vi "Sample_InputImpedance.vi"() -> ()   [LabVIEW 2013]
doc: "This samples demonstrates how to sample a finite waveform."
uses:
  <userlib>/ArtScope/Trigger/ArtScope_ConfigureTriggerSoftWare.vi
  <userlib>/ArtScope/Fetch/ArtScope_FetchBinary8.vi
  <userlib>/ArtScope/_SubVI/ArtScope_ArrayByChannel_U8.vi
panel:
  in  "bandwidth":i32(ring) items=["All"=-1, "Default"=0, "100M"=1, "20M"=2]
  in  "reference position":dbl
  in  "num samples":i32=1000
  in  "offset(mV)":i32
  in  "range(Vpp)":i32(ring) items=["20V", "10V", "2V", "40V", "16V", "8V", "4V", "1.6V", "800m", "400m", "160m", "80m", "40m"]
  in  "Stop":bool
  in  "input impendance":i32(ring) items=["1MΩ", "50Ω"]
  out "waveform":u8[][](graph)
  out "error out":errorcluster
  in  "timeout(s)":dbl=10.0
  in  "min record length":i32=1000
  in  "min sample rate":dbl=8000000.0
  in  "coupling":i32(ring) items=["DC", "AC"]
  in  "channel name":string="0"
  in  "resource name":string="Dev1"
  # "Vertical"
  # "Horizontal"
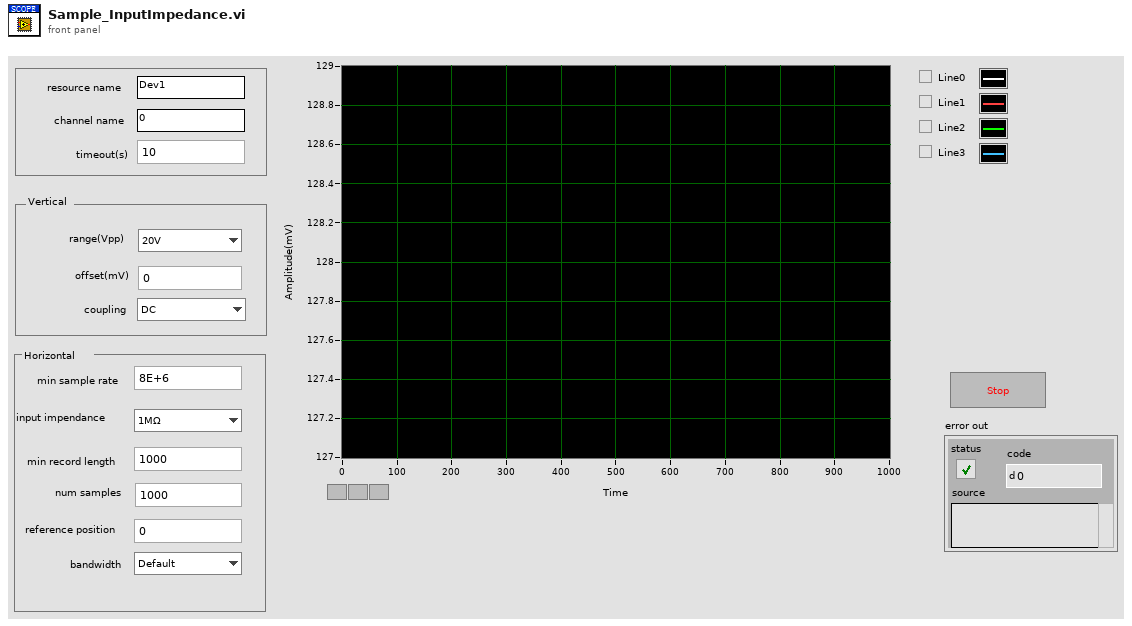
[diagram p1: front panel]
types:
  T1 = cluster{"fLSB":cluster{dbl, dbl, dbl, dbl, dbl, dbl, dbl, dbl}, "RangeValue":cluster{dbl, dbl, dbl, dbl, dbl, dbl, dbl, dbl}, "wMaxLSB":u32, "TriggerMode":i32, "sampLengthPerChan":u32, "pAvailSampsPoints":u32, "channelCount":i32}
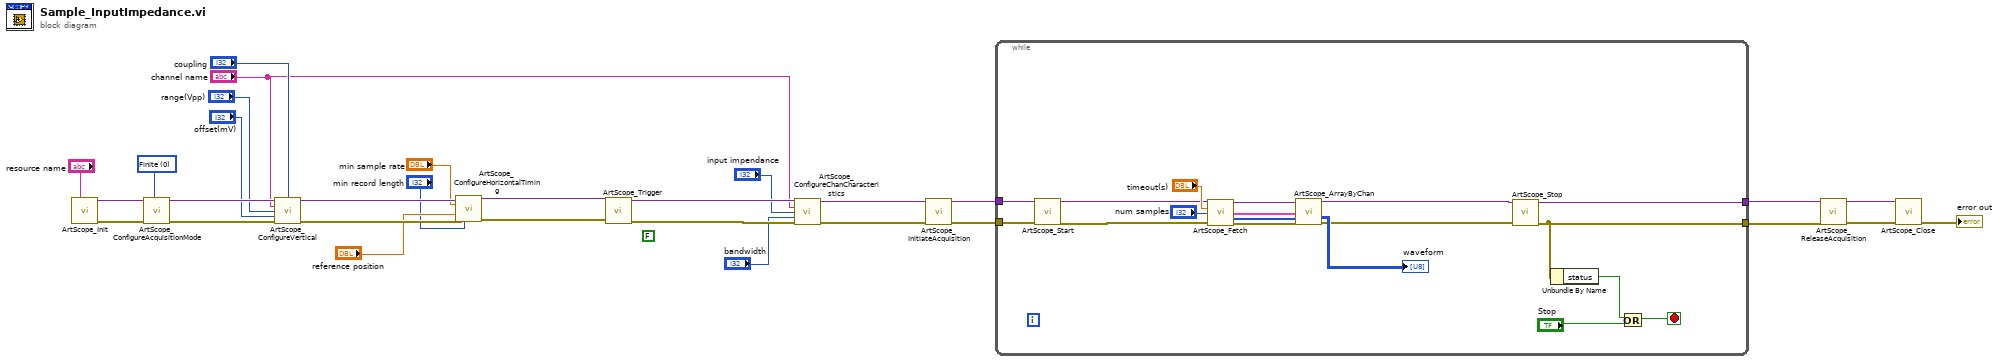
[diagram p0: block diagram]
diagram:
  (unwired) FALSE ("TrigOutEnable")
  w21 = 0 items=["Finite", "Continuous"] ("AcuqMode")
  n1 = call <userlib>:"ArtScope_Init.vi"("task name"="resource name") -> ("task handle"=w22:variant, "error out"=w23:errorcluster)  [unwired: 13 in]
  n2 = call <userlib>:"ArtScope_ConfigureAcquisitionMode.vi"("task handle"=w22, "acquisition mode"=w21, "error in (no error)"=w23) -> ("task handle"=w20:variant, "error out"=w24:errorcluster)  [unwired: 11 in]
  n3 = call <userlib>:"ArtScope_ConfigureVertical.vi"("task handle"=w20, "coupling"="coupling", "channels"="channel name", "range(Vpp)"="range(Vpp)", "offset"="offset(mV)", "error in (no error)"=w24) -> ("task handle"=w28:variant, "error out"=w27:errorcluster)  [unwired: 8 in]
  n4 = call <userlib>:"ArtScope_ConfigureHorizontalTiming.vi"("task handle"=w28, "min sample rate"="min sample rate", "reference position"="reference position", "error in (no error)"=w27, "min record length"="min record length") -> ("task handle"=w18:variant, "error out"=w19:errorcluster)  [unwired: 9 in]
  n5 = call-poly <userlib>:"ArtScope_Trigger.vi"("task handle"=w18, "error in (no error)"=w19) -> ("task handle"=w16:variant, "error out"=w15:errorcluster)  [unwired: 12 in]
  n6 = call <userlib>:"ArtScope_ConfigureChanCharacteristics.vi"("task handle"=w16, "channels"="channel name", "input impendence"="input impendance", "bandwidth"="bandwidth", "error in (no error)"=w15) -> ("task handle"=w11:variant, "error out"=w12:errorcluster)  [unwired: 9 in]
  n7 = call <userlib>:"ArtScope_InitiateAcquisition.vi"("task handle"=w11, "error in (no error)"=w12) -> ("task handle"=w6:variant, "error out"=w5:errorcluster)  [unwired: 12 in]
  n8 = while {
    tunnel: [w48] -> w7
    tunnel: [w44] -> w10
    tunnel: w6 -> [w45]
    tunnel: w5 -> [w46]
    stop <- w42 stop-if-true
    n9 = call <userlib>:"ArtScope_Start.vi"("task handle"=w45, "error in (no error)"=w46) -> ("task handle"=w40:variant, "error out"=w39:errorcluster)  [unwired: 12 in]
    n10 = call-poly <userlib>:"ArtScope_Fetch.vi"("task handle"=w40, "timeout"="timeout(s)", "num samples"="num samples", "error in (no error)"=w39) -> ("task handle"=w37:variant, "wfm info"=w35:T1, "data"=w34:u8[], "error out"=w36:errorcluster)  [unwired: 8 in]
    n11 = call-poly <userlib>:"ArtScope_ArrayByChan.vi"("task handle"=w37, "wfm info"=w35, "1D data"=w34, "error in (no error)"=w36) -> ("task handle"=w32:variant, "2D data"=→"waveform":u8[][], "error out"=w31:errorcluster)  [unwired: 9 in]
    n12 = call <userlib>:"ArtScope_Stop.vi"("task handle"=w32, "error in (no error)"=w31) -> ("task handle"=w48:variant, "error out"=w44:errorcluster)  [unwired: 12 in]
    n13 = Unbundle By Name(w44) -> ("status"=w43:bool)
    n14 = Or(x=w43, y="Stop") -> (x .or. y?=w42:bool)
  }
  n15 = call <userlib>:"ArtScope_ReleaseAcquisition.vi"("task handle"=w7, "error in (no error)"=w10) -> ("task handle"=w8:variant, "error out"=w9:errorcluster)  [unwired: 12 in]
  n16 = call <userlib>:"ArtScope_Close.vi"("task handle"=w8, "error in (no error)"=w9) -> ("error out"=→"error out":errorcluster)  [unwired: 13 in]
